vi "Write to Flashcard to CSV.vi"(8 "error in":errorcluster, 9 "DATA":T1(array[cluster]), 10 "Columns":string[](array[string]), 11 "stripped path":path) -> (0 "error out":errorcluster, 3 "actual path":path)   [LabVIEW 2019, in "flashcards.lvlib"]
uses:
  flashcards.lvlib
  <vilib>/Utility/sysdir.llb/System Directory Type.ctl
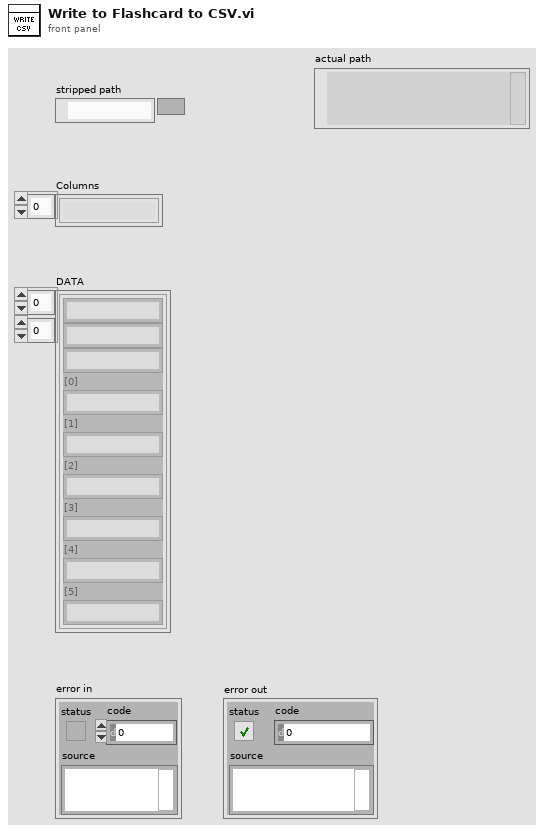
[diagram p1: front panel]
types:
  T1 = cluster{string, string, string, "[0]":string, "[1]":string, "[2]":string, "[3]":string, "[4]":string, "[5]":string}[][]
  T2 = typedef "System Directory Type.ctl" = i32
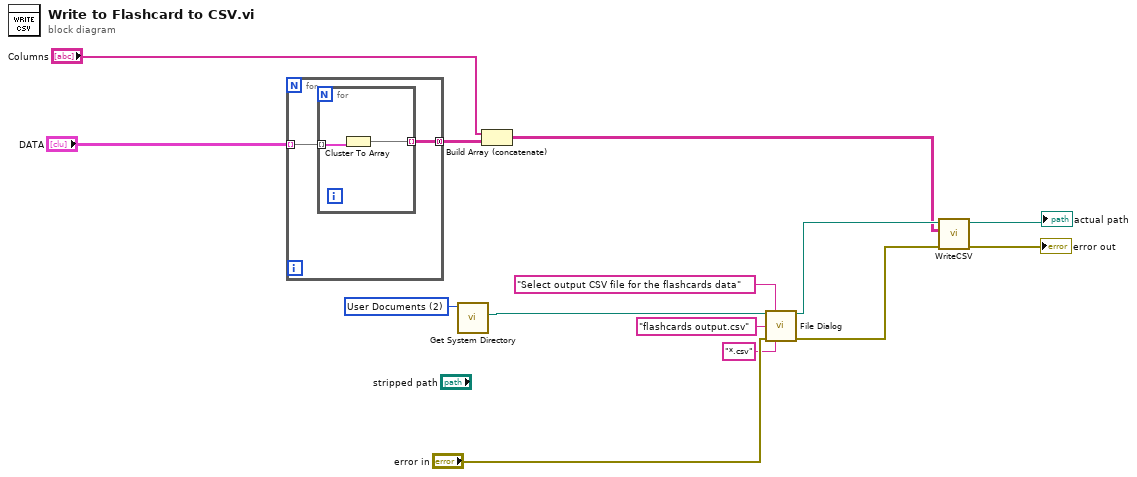
[diagram p0: block diagram]
diagram:
  w6 = T2 2 items=["User Home"=0, "User Desktop"=1, "User Documents"=2, "User Application Data"=3, "User Preferences"=4, "User Temporary"=5, "Public Documents"=6, "Public Application Data"=7, "Public Preferences"=8, "Public Cache"=13, "System Core Libraries"=9, "System Installed Libraries"=10, "Application Files"=11, "Boot Volume Root"=12] ("system directory type")
  n1 = for {
    tunnel: "DATA" -> [w16] mode=indexing
    tunnel: [w15] -> w13 mode=concatenating
    n2 = for {
      tunnel: w16 -> [w18] mode=indexing
      tunnel: [w17] -> w15 mode=indexing
      n3 = Cluster To Array(cluster=w18) -> (array=w17:string[])
    }
  }
  n4 = call <vilib>:"Get System Directory.vi"("system directory type"=w6) -> ("system directory"=w5:path)  [unwired: 10 in]
  n5 = Build Array (concatenate)("Columns", w13) -> (w3:string[][])
  n6 = call "File Dialog"("start path"=w5, "prompt"="Select output CSV file for the flashcards data", "default name"="flashcards output.csv", "error in"="error in", "pattern (all files)"="*.csv") -> ("selected path"=w4:path, "error out"=w9:errorcluster)  [unwired: 7 in, 2 out]
  n7 = call "WriteCSV.vi"("error in (no error)"=w9, "Data to Write"=w3, "file path (empty creates file in temp folder)"=w4) -> ("error out"=→"error out":errorcluster, "actual path"=→"actual path":path)  [unwired: 7 in]
